vi "ClsShowSpectrum.vi"(8 "error in (no error)":errorcluster, 11 "Connection Out in":u32) -> (0 "error out":errorcluster, 3 "Connection Out out":u32)   [LabVIEW 2015]
uses:
  TypeDefs/ClsConfigureValues.ctl
  TypeDefs/ClsCommandOrder.ctl
  ClsSendCmds_Array.vi
panel:
  in  "Tab Control":T1(tab)
  out "Spectrum of Multiple Channels 2":i16[][](graph)
  in  "Map Selector 2":T2(ring)=enum."original"
  out "Waveform Graph":i16[](graph)
  in  "Channelselect":i32
  out "Line Profile":dbl[](graph)
  in  "Subtract Reference?":bool
  in  "White Reference":bool
  in  "Dark Reference":bool
  in  "Load Config":bool
  out "Command Response":string
  in  "Command":string
  in  "ClsConfigureValues":T3
  in  "stop":bool
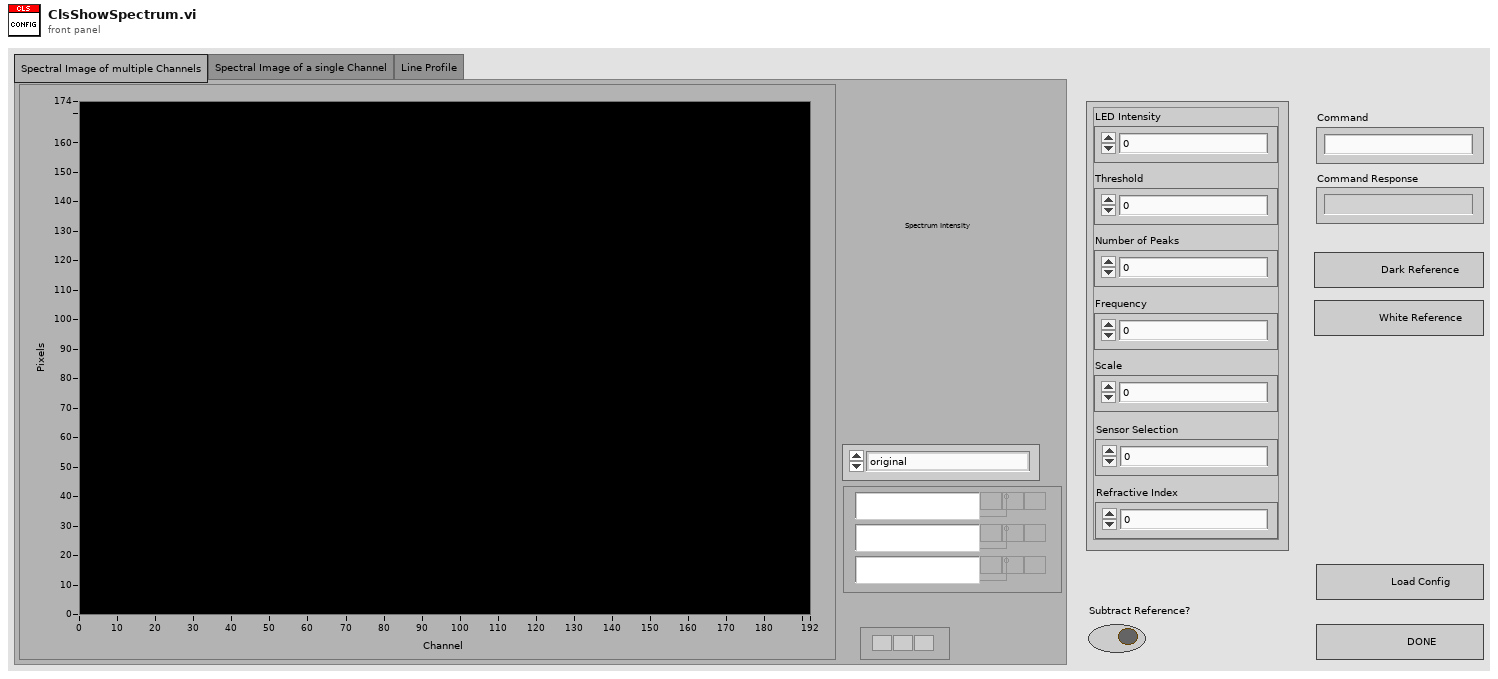
[diagram p1: front panel]
types:
  T1 = enum32{"Spectral Image of multiple Channels", "Spectral Image of a single Channel", "Line Profile"}
  T2 = enum16{"fire", "rainbow", "gray", "inverse gray", "ice", "original"}
  T3 = typedef "ClsConfigureValues.ctl" = cluster{"LED Intensity":dbl, "Threshold":dbl, "Number of Peaks":dbl, "Frequency":dbl, "Scale":dbl, "Sensor Selection":dbl, "Refractive Index":dbl}
  T4 = typedef "ClsCommandOrder.ctl" = string[]
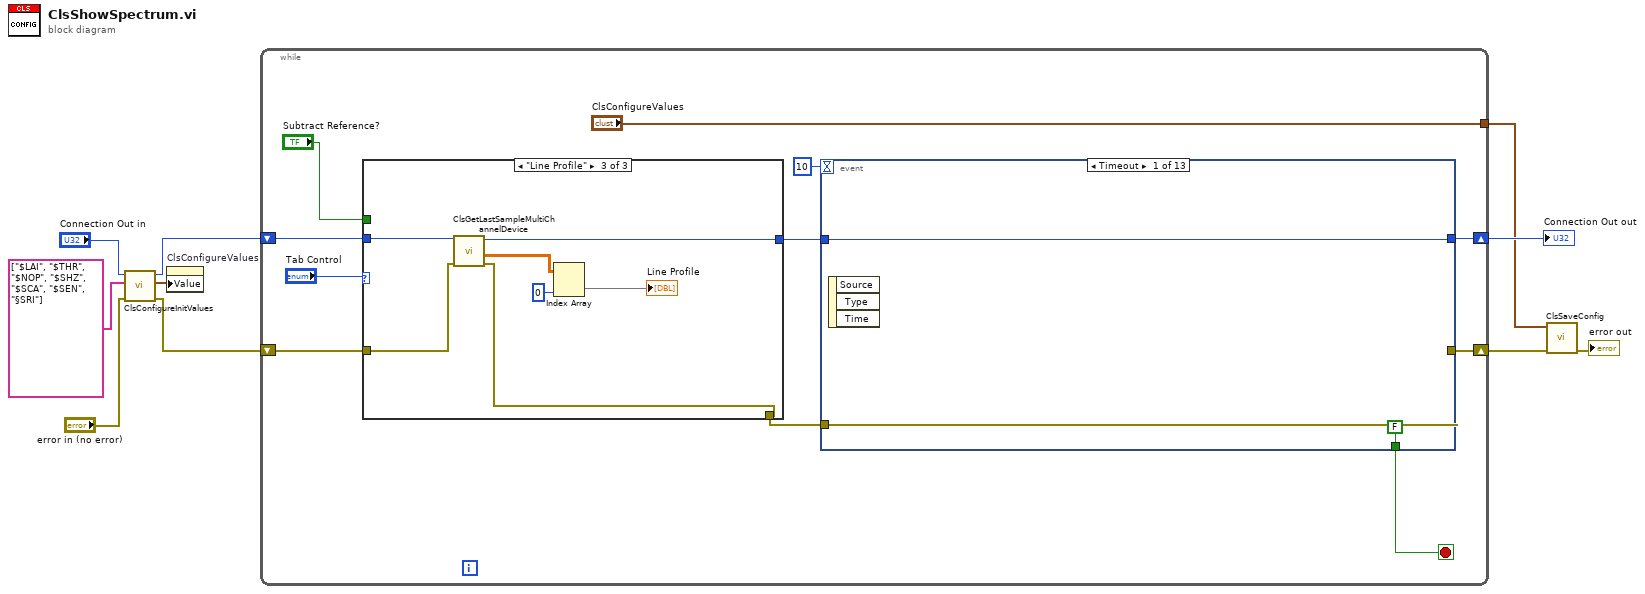
[diagram p0: block diagram]
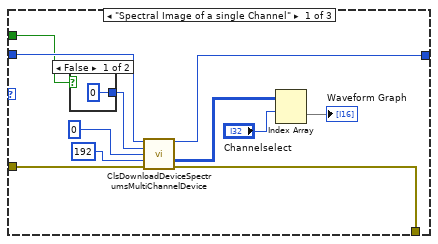
[diagram p2: hidden frame]
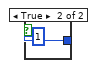
[diagram p3: hidden frame]
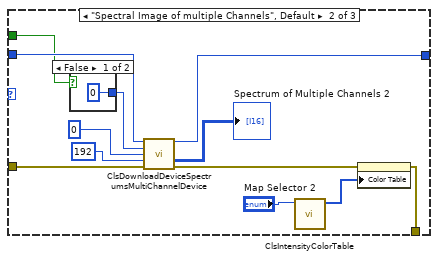
[diagram p4: hidden frame]
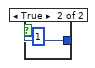
[diagram p5: hidden frame]
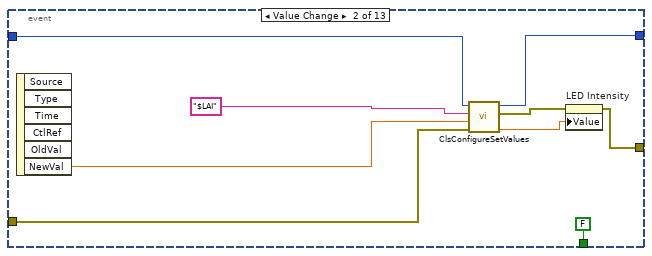
[diagram p6: hidden frame]
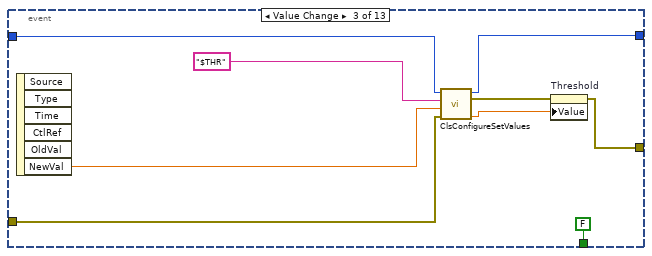
[diagram p7: hidden frame]
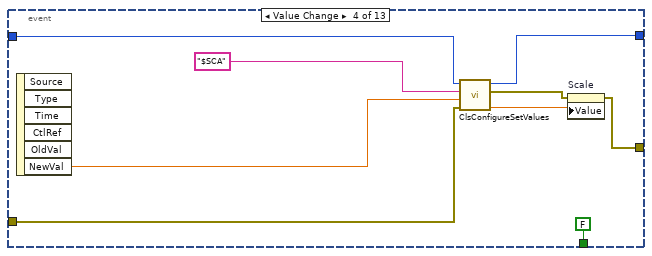
[diagram p8: hidden frame]
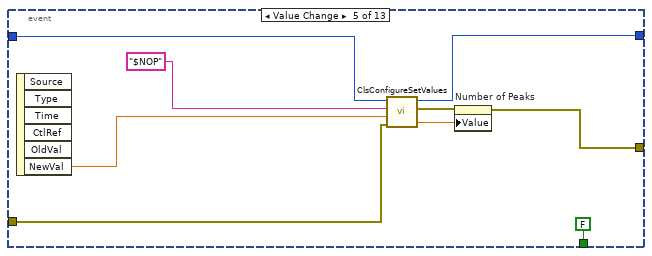
[diagram p9: hidden frame]
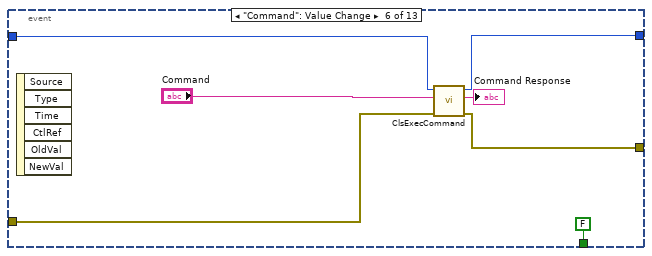
[diagram p10: hidden frame]
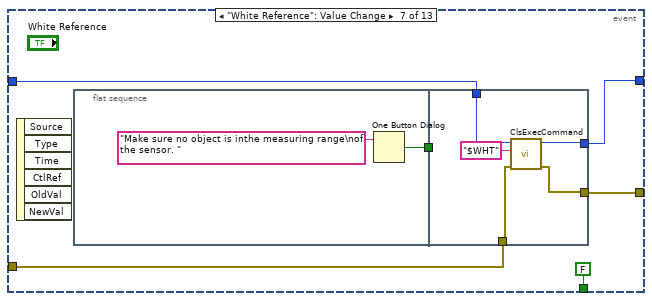
[diagram p11: hidden frame]
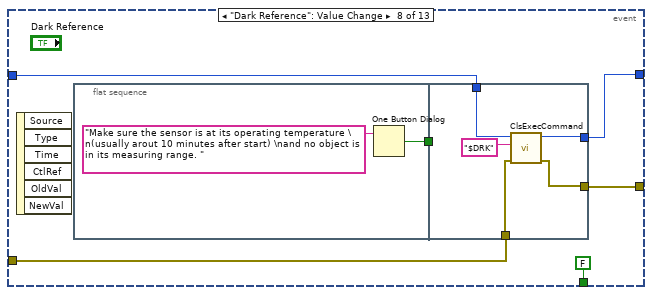
[diagram p12: hidden frame]
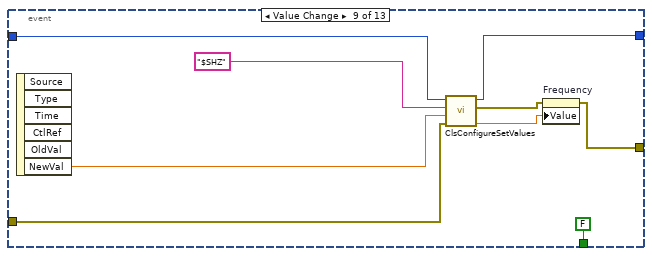
[diagram p13: hidden frame]
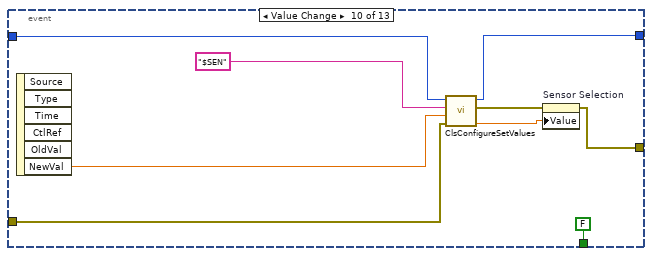
[diagram p14: hidden frame]
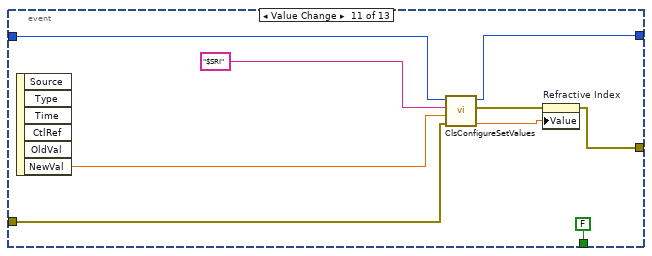
[diagram p15: hidden frame]
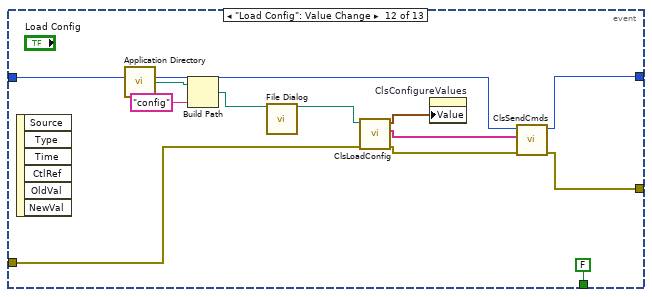
[diagram p16: hidden frame]
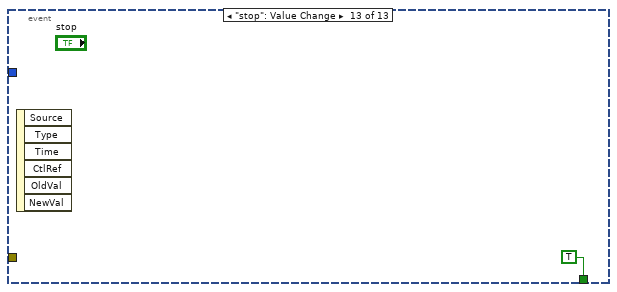
[diagram p17: hidden frame]
diagram:
  n1 = call "ClsConfigureInitValues.vi"("error in (no error)"="error in (no error)", "InitCommandArray"=T4 ["$LAI", "$THR", "$NOP", "$SHZ", "$SCA", "$SEN", "§SRI"], "Connection Out in in"="Connection Out in") -> ("error out"=w5:errorcluster, "out"=w4:T3, "Connection Out out 2"=w8:u32)  [unwired: 6 in]
  n2 = property on="ClsConfigureValues" class="Clust (strict)"("Value"=w4) -> ()  [unwired: 2 in, 2 out]
  n3 = while {
    shift-right: [w16] -> w3
    shift-left: w5 -> [w20]
    shift-right: [w18] -> w10
    shift-left: w8 -> [w21]
    tunnel: ["ClsConfigureValues"] -> w1
    stop <- w13 stop-if-true
    n4 = case shown="\"Line Profile\"" "Tab Control" {
      tunnel: w21 -> [w32 w43 w55]
      tunnel: w20 -> [w31 w42 w53]
      tunnel: [w30 w41 w54] -> w19
      tunnel: [w22 w40 w52] -> w15
      tunnel: "Subtract Reference?" -> [w26 w35 _]
      frame "Spectral Image of a single Channel" {
        n5 = case shown="False" w26 {
          tunnel: [0 ("Spectrum Type") 1 ("Spectrum Type")] -> w29
          frame False {
          }
          frame True {
          }
        }
        n6 = call "ClsDownloadDeviceSpectrumsMultiChannelDevice.vi"("Connection In"=w32, "Spectrum Type"=w29, "Start Channel Index"=0, "Number of Channels"=192, "error in (no error)"=w31) -> ("Connection Out"=w30:u32, "Spectrums"=w24:i16[][], "error out"=w22:errorcluster)  [unwired: 8 in]
        n7 = Index Array(array=w24, index (row)="Channelselect") -> (element=→"Waveform Graph":i16[])  [unwired: 1 in]
      }
      frame "Spectral Image of multiple Channels", Default {
        n8 = case shown="False" w35 {
          tunnel: [0 ("Spectrum Type") 1 ("Spectrum Type")] -> w39
          frame False {
          }
          frame True {
          }
        }
        n9 = call "ClsDownloadDeviceSpectrumsMultiChannelDevice.vi"("Connection In"=w43, "Spectrum Type"=w39, "Start Channel Index"=0, "Number of Channels"=192, "error in (no error)"=w42) -> ("Connection Out"=w41:u32, "Spectrums"=→"Spectrum of Multiple Channels 2":i16[][], "error out"=w46:errorcluster)  [unwired: 8 in]
        n10 = call "ClsIntensityColorTable.vi"("Map Selector"="Map Selector 2") -> ("Color Map Array"=w45:u32[])  [unwired: 10 in]
        n11 = property on="Spectrum of Multiple Channels 2" class="IntGraph (strict)"(error in=w46, "Color Table"=w45) -> (error out=w40:errorcluster)  [unwired: 1 in, 1 out]
      }
      frame "Line Profile" {
        n12 = call "ClsGetLastSampleMultiChannelDevice.vi"("error in"=w53, "Connection In"=w55) -> ("error out"=w52:errorcluster, "Peak Signals"=w51:dbl[][], "Connection Out"=w54:u32)  [unwired: 5 in, 2 out]
        n13 = Index Array(array=w51, index (col)=0 ("disabled index (col)")) -> (element=→"Line Profile":dbl[])  [unwired: 1 in]
      }
    }
    n14 = event shown="[0] Timeout" {
      selector: _ -> [_ _ _ _ _ _ _ _ _ _ _ _ _]
      dyn-events: _ -> [_ _ _ _ _ _ _ _ _ _ _ _ _]
      timeout: 10 -> [_ _ _ _ _ _ _ _ _ _ _ _ _]
      tunnel: w19 -> [w58 w65 w76 w85 w94 w100 w107 w120 w136 w145 w154 w160 _]
      tunnel: [w58 w64 w69 w81 w92 w99 w106 w119 w130 w139 w148 w161 _] -> w18
      tunnel: [w57 w60 w70 w78 w89 w97 w104 w117 w129 w138 w147 w162 _] -> w16
      tunnel: w15 -> [w57 w67 w73 w83 w91 w98 w105 w118 w133 w142 w151 w166 _]
      tunnel: [FALSE FALSE FALSE FALSE FALSE FALSE FALSE FALSE FALSE FALSE FALSE FALSE TRUE] -> w13
      event Timeout {
        n15 = event-data() -> ()  [unwired: 1 in, 3 out]
      }
      event Value Change {
        n16 = event-data() -> ("NewVal"=w63:dbl)  [unwired: 1 in, 5 out]
        n17 = call "ClsConfigureSetValues.vi"("error in (no error)"=w67, "NewVal"=w63, "string"="$LAI", "Connection Out in"=w65) -> ("Response"=w62:dbl, "error out"=w61:errorcluster, "Connection Out out"=w64:u32)  [unwired: 5 in]
        n18 = property on="LED Intensity" class="DigNum (strict)"(error in=w61, "Value"=w62) -> (error out=w60:errorcluster)  [unwired: 1 in, 1 out]
      }
      event Value Change {
        n19 = event-data() -> ("NewVal"=w74:dbl)  [unwired: 1 in, 5 out]
        n20 = call "ClsConfigureSetValues.vi"("error in (no error)"=w73, "NewVal"=w74, "string"="$THR", "Connection Out in"=w76) -> ("Response"=w72:dbl, "error out"=w71:errorcluster, "Connection Out out"=w69:u32)  [unwired: 5 in]
        n21 = property on="Threshold" class="DigNum (strict)"(error in=w71, "Value"=w72) -> (error out=w70:errorcluster)  [unwired: 1 in, 1 out]
      }
      event Value Change {
        n22 = event-data() -> ("NewVal"=w82:dbl)  [unwired: 1 in, 5 out]
        n23 = call "ClsConfigureSetValues.vi"("error in (no error)"=w83, "NewVal"=w82, "string"="$SCA", "Connection Out in"=w85) -> ("Response"=w80:dbl, "error out"=w79:errorcluster, "Connection Out out"=w81:u32)  [unwired: 5 in]
        n24 = property on="Scale" class="DigNum (strict)"(error in=w79, "Value"=w80) -> (error out=w78:errorcluster)  [unwired: 1 in, 1 out]
      }
      event Value Change {
        n25 = event-data() -> ("NewVal"=w90:dbl)  [unwired: 1 in, 5 out]
        n26 = call "ClsConfigureSetValues.vi"("error in (no error)"=w91, "NewVal"=w90, "string"="$NOP", "Connection Out in"=w94) -> ("Response"=w87:dbl, "error out"=w88:errorcluster, "Connection Out out"=w92:u32)  [unwired: 5 in]
        n27 = property on="Number of Peaks" class="DigNum (strict)"(error in=w88, "Value"=w87) -> (error out=w89:errorcluster)  [unwired: 1 in, 1 out]
      }
      event "Command": Value Change {
        n28 = event-data() -> ()  [unwired: 1 in, 6 out]
        n29 = call "ClsExecCommand.vi"("error in (no error)"=w98, "Command In"="Command", "Connection In"=w100) -> ("error out"=w97:errorcluster, "Command Response"=→"Command Response":string, "Connection Out"=w99:u32)  [unwired: 6 in]
      }
      event "White Reference": Value Change {
        n30 = event-data() -> ()  [unwired: 1 in, 6 out]
        n31 = flat-sequence {
          tunnel: [w108] -> w103
          tunnel: w107 -> [w113]
          tunnel: [w112] -> w106
          tunnel: w105 -> [w111]
          tunnel: [w110] -> w104
          tunnel: w103 -> [_]
          frame #0 {
            n32 = One Button Dialog(message="Make sure no object is inthe measuring range\nof the sensor. ") -> (true=w108:bool)  [unwired: 1 in]
          }
          frame #1 {
            n33 = call "ClsExecCommand.vi"("error in (no error)"=w111, "Command In"="$WHT", "Connection In"=w113) -> ("error out"=w110:errorcluster, "Connection Out"=w112:u32)  [unwired: 6 in, 1 out]
          }
        }
      }
      event "Dark Reference": Value Change {
        n34 = event-data() -> ()  [unwired: 1 in, 6 out]
        n35 = flat-sequence {
          tunnel: [w121] -> w116
          tunnel: w120 -> [w126]
          tunnel: [w125] -> w119
          tunnel: w118 -> [w124]
          tunnel: [w123] -> w117
          tunnel: w116 -> [_]
          frame #0 {
            n36 = One Button Dialog(message="Make sure the sensor is at its operating temperature \n(usually arout 10 minutes after start) \nand no object is in its measuring range. ") -> (true=w121:bool)  [unwired: 1 in]
          }
          frame #1 {
            n37 = call "ClsExecCommand.vi"("error in (no error)"=w124, "Command In"="$DRK", "Connection In"=w126) -> ("error out"=w123:errorcluster, "Connection Out"=w125:u32)  [unwired: 6 in, 1 out]
          }
        }
      }
      event Value Change {
        n38 = event-data() -> ("NewVal"=w134:dbl)  [unwired: 1 in, 5 out]
        n39 = call "ClsConfigureSetValues.vi"("error in (no error)"=w133, "NewVal"=w134, "string"="$SHZ", "Connection Out in"=w136) -> ("Response"=w132:dbl, "error out"=w131:errorcluster, "Connection Out out"=w130:u32)  [unwired: 5 in]
        n40 = property on="Frequency" class="DigNum (strict)"(error in=w131, "Value"=w132) -> (error out=w129:errorcluster)  [unwired: 1 in, 1 out]
      }
      event Value Change {
        n41 = event-data() -> ("NewVal"=w143:dbl)  [unwired: 1 in, 5 out]
        n42 = call "ClsConfigureSetValues.vi"("error in (no error)"=w142, "NewVal"=w143, "string"="$SEN", "Connection Out in"=w145) -> ("Response"=w141:dbl, "error out"=w140:errorcluster, "Connection Out out"=w139:u32)  [unwired: 5 in]
        n43 = property on="Sensor Selection" class="DigNum (strict)"(error in=w140, "Value"=w141) -> (error out=w138:errorcluster)  [unwired: 1 in, 1 out]
      }
      event Value Change {
        n44 = event-data() -> ("NewVal"=w152:dbl)  [unwired: 1 in, 5 out]
        n45 = call "ClsConfigureSetValues.vi"("error in (no error)"=w151, "NewVal"=w152, "string"="$SRI", "Connection Out in"=w154) -> ("Response"=w150:dbl, "error out"=w149:errorcluster, "Connection Out out"=w148:u32)  [unwired: 5 in]
        n46 = property on="Refractive Index" class="DigNum (strict)"(error in=w149, "Value"=w150) -> (error out=w147:errorcluster)  [unwired: 1 in, 1 out]
      }
      event "Load Config": Value Change {
        n47 = event-data() -> ()  [unwired: 1 in, 6 out]
        n48 = call <vilib>:"Application Directory.vi"() -> ("Application Directory"=w157:path)
        n49 = Build Path(base path=w157, name or relative path="config") -> (appended path=w159:path)
        n50 = call "File Dialog"("start path"=w159) -> ("selected path"=w156:path)  [unwired: 11 in, 3 out]
        n51 = call "ClsLoadConfig.vi"("error in (no error)"=w166, "XML File Path"=w156) -> ("error out"=w164:errorcluster, "ClsCondigureValues (Array)"=w165:string[], "ClsConfigureValues (Cluster)"=w163:T3)  [unwired: 7 in]
        n52 = property on="ClsConfigureValues" class="Clust (strict)"("Value"=w163) -> ()  [unwired: 2 in, 2 out]
        n53 = call-poly "ClsSendCmds.vi"("error in (no error)"=w164, "InitCommandArray"=w165, "Connection Out in"=w160) -> ("error out"=w162:errorcluster, "Connection Out out"=w161:u32)  [unwired: 6 in, 1 out]
      }
      event "stop": Value Change {
        n54 = event-data() -> ()  [unwired: 1 in, 6 out]
      }
    }
  }
  "Connection Out out" <- w10
  n55 = call "ClsSaveConfig.vi"("error in (no error)"=w3, "ClsConfigureValues"=w1) -> ("error out"=→"error out":errorcluster)  [unwired: 9 in]
